vi "ADIS16470 Read.vi"(8 "error in (no error)":errorcluster, 11 "ADIS16470DevRef":T2) -> (0 "error out":errorcluster, 1 "ADIS16470 Buffer":T1[](array[typedef]), 2 "ADIS16470 Value":T1, 3 "ADIS16470DevRef":T2)   [LabVIEW 2018]
uses:
  Typedef/ADIS16470 Device Reference.ctl
  Typedef/ADIS16470 Hardware Configuration.ctl
  <vilib>/Rock Robotics/WPI/SPI/WPI_SPIMode.ctl
  <vilib>/Rock Robotics/SystemInterfaces/DIO/FPGA_DIOChannel.ctl
  <vilib>/Rock Robotics/SystemInterfaces/spilib/spi_bus.ctl
  Typedef/ADIS16470 Data.ctl
  Typedef/ADIS16470 Status.ctl
  Typedef/ADIS16470 Process.ctl
  Typedef/ADIS16470 Command Type.ctl
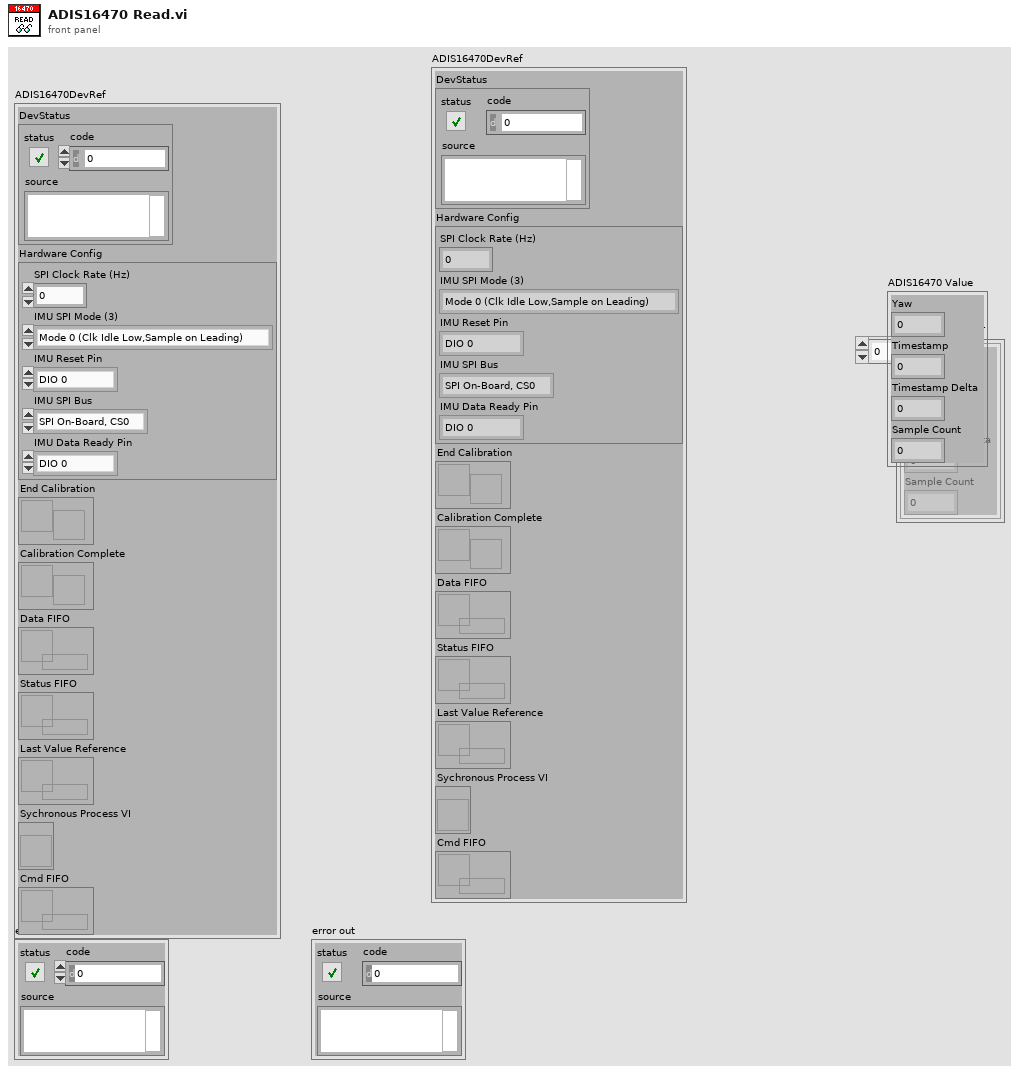
[diagram p1: front panel]
types:
  T1 = typedef "ADIS16470 Data.ctl" = cluster{"Yaw":dbl, "Timestamp":dbl, "Timestamp Delta":dbl, "Sample Count":u16}
  T2 = typedef "ADIS16470 Device Reference.ctl" = cluster{"DevStatus":errorcluster, "Hardware Config":T3, "End Calibration":refnum<notifier>, "Calibration Complete":refnum<notifier>, "Data FIFO":refnum<k33>, "Status FIFO":refnum<k33>, "Last Value Reference":refnum<data-value>, "Sychronous Process VI":T7, "Cmd FIFO":refnum<k33>}
  T3 = typedef "ADIS16470 Hardware Configuration.ctl" = cluster{"SPI Clock Rate (Hz)":dbl, "IMU SPI Mode (3)":T4, "IMU Reset Pin":T5, "IMU SPI Bus":T6, "IMU Data Ready Pin":T5}
  T4 = typedef "WPI_SPIMode.ctl" = enum16{"Mode 0 (Clk Idle Low,Sample on Leading)", "Mode 1 (Clk Idle Low,Sample on Trailing)", "Mode 2 (Clk Idle High,Sample on Leading)", "Mode 3 (Clk Idle High,Sample on Trailing)"}
  T5 = typedef "FPGA_DIOChannel.ctl" = enum8{"DIO 0", "DIO 1", "DIO 2", "DIO 3", "DIO 4", "DIO 5", "DIO 6", "DIO 7", "DIO 8", "DIO 9", "DIO MXP 0", "DIO MXP 1", "DIO MXP 2", "DIO MXP 3", "DIO MXP 4", "DIO MXP 5", "DIO MXP 6", "DIO MXP 7", "DIO MXP 8", "DIO MXP 9", "DIO MXP 10", "DIO MXP 11", "DIO MXP 12", "DIO MXP 13", "DIO MXP 14", "DIO MXP 15", "SPI Port CS1", "SPI Port CS2", "SPI Port CS3", "SPI Port MISO", "SPI Port MOSI", "Invalid"}
  T6 = typedef "spi_bus.ctl" = enum16{"SPI On-Board, CS0", "SPI On-Board, CS1", "SPI On-Board, CS2", "SPI On-Board, CS3", "SPI MXP", "Invalid"}
  T7 = typedef "ADIS16470 Process.ctl" = refnum<vi>
  T8 = typedef "ADIS16470 Status.ctl" = cluster{"Calibrated?":bool}
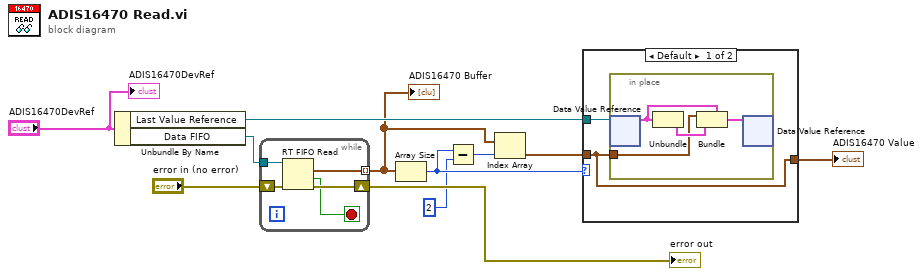
[diagram p0: block diagram]
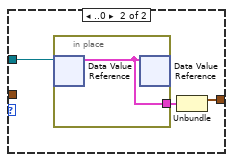
[diagram p2: hidden frame]
diagram:
  n1 = Unbundle By Name("ADIS16470DevRef") -> ("Last Value Reference"=w8:refnum<data-value>, "Data FIFO"=w10:refnum<k33>)
  n2 = while {
    tunnel: w10 -> [w15]
    tunnel: [w12] -> w2 mode=indexing
    shift-right: [w14] -> w7
    shift-left: "error in (no error)" -> [w16]
    stop <- w13 stop-if-true
    n3 = RT FIFO Read(0:w15, 3:w16) -> (9:w12:T1, 10:w13:bool, 11:w14:errorcluster)  [unwired: 2 in, 2 out]
  }
  "error out" <- w7
  "ADIS16470 Buffer" <- w2
  n4 = Array Size(array=w2) -> (size(s)=w5:i32)
  n5 = Subtract(x=w5, y=2 ("x")) -> (x-y=w3:i32)
  n6 = Index Array(array=w2, index=w3) -> (element=w1:T1)
  n7 = case shown="Default" w5 {
    tunnel: w8 -> [w18 w25]
    tunnel: w1 -> [w17 _]
    tunnel: [w17 w23] -> w6
    frame Default {
      n8 = in-place {
        in-place-border: w17 -> [w19]
        n9 = in-place-dvr #1(w18) -> (w21:cluster{T1, T8})  [unwired: 1 out]
        n10 = Unbundle(w21) -> (w20:T8)  [unwired: 1 out]
        n11 = Bundle(cluster=w21, w19, w20) -> (w22:cluster{T1, T8})
        n12 = in-place-dvr #1(w22) -> ()  [unwired: 2 out]
      }
    }
    frame ..0 {
      n13 = in-place {
        in-place-border: [w26] -> w24
        n14 = in-place-dvr #2(w25) -> (w26:cluster{T1, T8})  [unwired: 1 out]
        n15 = in-place-dvr #2(w26) -> ()  [unwired: 2 out]
      }
      n16 = Unbundle(w24) -> (w23:T1)  [unwired: 1 out]
    }
  }
  "ADIS16470 Value" <- w6
  "ADIS16470DevRef" <- "ADIS16470DevRef"
